vi "recalculate valubility.vi"(0 "valubility":dbl[][](array[numeric]), 1 "teams in match":i16[](array[numeric]), 2 "median":dbl=1.0, 3 "team number":i16, 4 "scores":i16[](array[numeric])) -> (6 "team in match?":bool, 7 "valubility":dbl[](array[numeric]))   [LabVIEW 2009]
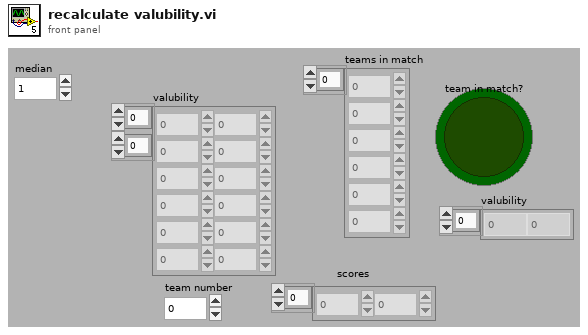
[diagram p1: front panel]
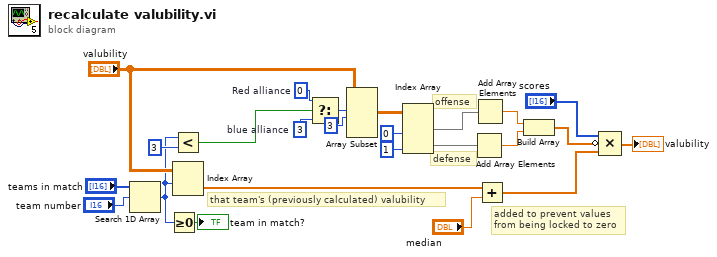
[diagram p0: block diagram]
diagram:
  w13 = 3  # blue alliance
  w14 = 0  # Red alliance
  # "added to prevent values from being locked to zero"
  # "that team's (previously calculated) valubility"
  # "defense"
  # "offense"
  n1 = Search 1D Array(1D array="teams in match", element="team number") -> (index of element=w5:i32)  [unwired: 1 in]
  n2 = Greater Or Equal To 0?(x=w5) -> (x >= 0?=→"team in match?":bool)
  n3 = Less?(x=w5, y=3) -> (x < y?=w12:bool)
  n4 = Index Array(array="valubility", index (row)=w5) -> (element=w2:dbl[])  [unwired: 1 in]
  n5 = Select(t=w14, s=w12, f=w13) -> (s? t:f=w15:i32)
  n6 = Array Subset(array="valubility", index (row)=w15, length (row)=3 ("length")) -> (w23:dbl[][])  [unwired: 2 in]
  n7 = Index Array(array=w23, index (col) #1=0 ("disabled index (col)"), index (col) #2=1 ("index (col)")) -> (element #1=w19:dbl[], element #2=w18:dbl[])  [unwired: 2 in]
  n8 = Add Array Elements(numeric array=w18) -> (sum=w16:dbl)
  n9 = Add Array Elements(numeric array=w19) -> (sum=w17:dbl)
  n10 = Add(x=w2, y="median") -> (x+y=w1:dbl[])
  n11 = Build Array(w17, w16) -> (w11:dbl[])
  n12 = Compound Arithmetic op=MULTIPLY("scores", invert w11, w1) -> (→"valubility":dbl[])
